vi "VT4001_Chamber Test.vi"(8 "error in":errorcluster, 10 "Target Temp(°C)":dbl=25.0, 11 "COM VISA Resource":refnum<visa-resource-name>="COM6") -> (0 "error out":errorcluster, 2 "OK":bool=TRUE)   [LabVIEW 2019]
doc: "Modbus Comm Tester\n\nThis VI demonstrates the usage of the Modbus Master API for both TCP and Serial connections.\nIt is also a useful tool for testing communication with your modbus device. You can test different\ncommunication parameters and coil/register address ranges without having to write any code.\n\nCopyright (c) 2016, Plasmionique Inc.\nAll rights reserved.\n\nLicense: BSD (2-Clause) - http://opensource.org/licenses/BSD-2-Clause"
uses:
  <vilib>/Plasmionique/MB Master/MB_Master_Serial/MB_Master_Serial.lvclass
  D:/National Instruments/LabVIEW 2019/vi.lib/Plasmionique/MB Master/MB_Master/MB_Master.lvclass
  <vilib>/Plasmionique/MB Master/MB Master.lvlib
panel:
  out "Numeric":i32
  out "Temp Read":u16
  # "Communication Settings"
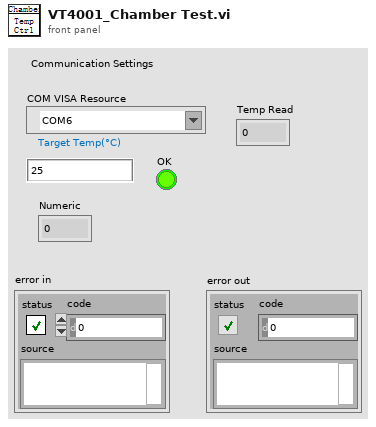
[diagram p1: front panel]
types:
  T1 = cluster{"baud rate (bps)":u32, "stop bits":u16, "parity":u16, "flow control":u16, "timeout":u32, "retries":i32}
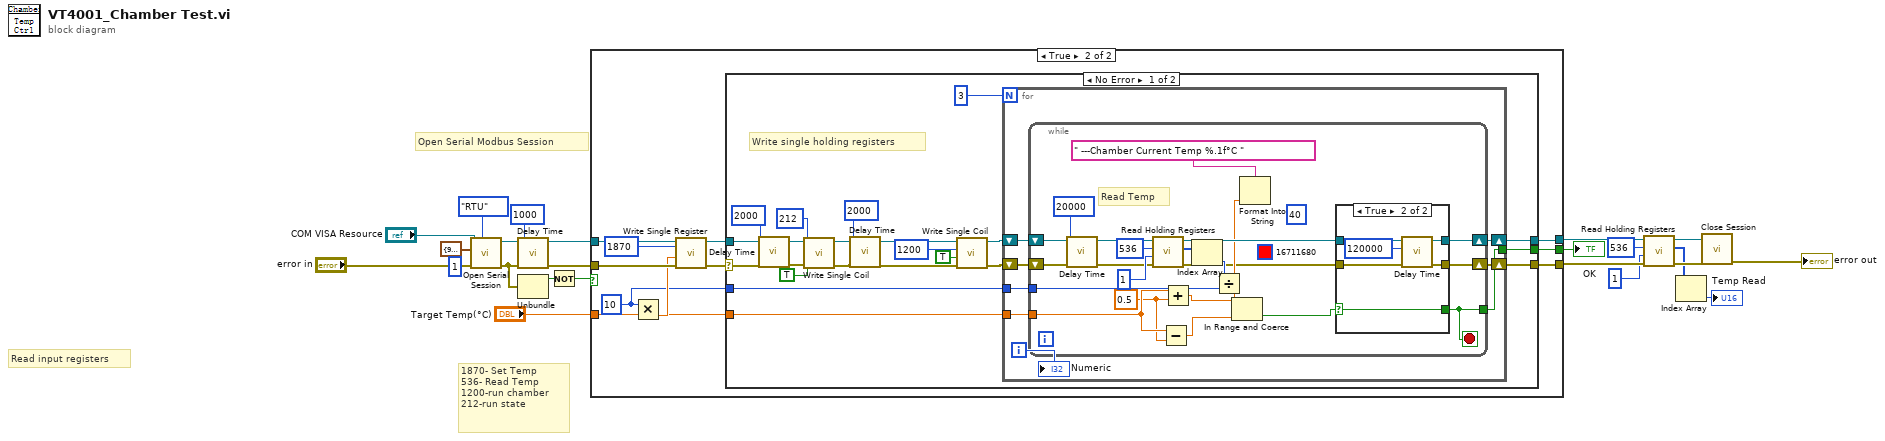
[diagram p0: block diagram]
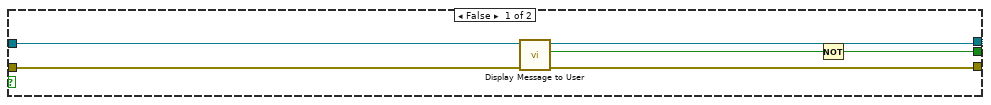
[diagram p2: hidden frame]
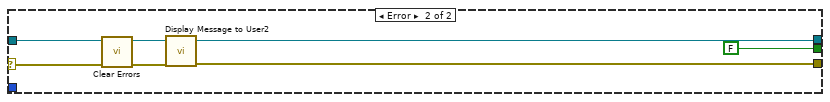
[diagram p4: hidden frame]
diagram:
  # "Open Serial Modbus Session"
  # "1870- Set Temp\n536- Read Temp\n1200-run chamber\n212-run state"
  # "Read input registers"
  n1 = call <vilib>:"Open Serial Session.vi"("Mode (RTU)"=enum16{"RTU", "ASCII"}."RTU", "Error in"="error in", "Slave ID"=u8 1, "Serial Config"=T1 {"baud rate (bps)"=9600, "stop bits"=10, "parity"=0, "flow control"=0, "timeout"=1000, "retries"=1}, "VISA Resource"="COM VISA Resource") -> ("Error out"=w19:errorcluster, "MB_Serial session"=w20:refnum<class "MB_Master_Serial.lvclass">)  [unwired: 5 in]
  n2 = call "Delay Time.vi"("Error In"=w19, "Delay Time (ms)"=u32 1000) -> ("Error Out"=w18:errorcluster)  [unwired: 9 in]
  n3 = Unbundle(w19) -> ("status"=w22:bool)  [unwired: 2 out]
  n4 = Not(x=w22) -> (.not. x?=w21:bool)
  n5 = case shown="True" w21 {
    tunnel: w20 -> [w23 w38]
    tunnel: w18 -> [w27 w37]
    tunnel: "Target Temp(°C)" -> [_ w29]
    tunnel: [w26 w36] -> w8
    tunnel: [w24 w35] -> w17
    tunnel: [w23 w34] -> w7
    frame False {
      n6 = call "Display Message to User"("error in (no error)"=w27) -> ("error out"=w26:errorcluster, "OK"=w25:bool)  [unwired: 9 in]
      n7 = Not(x=w25) -> (.not. x?=w24:bool)
    }
    frame True {
      w30 = u16 10 ("x")
      n8 = Multiply(x=w30, y=w29) -> (x*y=w31:dbl)
      n9 = call <vilib>:"Write Single Register.vi"("error in (no error)"=w37, "value"=w31, "address"=u16 1870, "MB session in"=w38) -> ("error out"=w28:errorcluster, "MB session out"=w32:refnum<class "MB_Master_Serial.lvclass">)  [unwired: 6 in]
      n10 = case shown="No Error" w28 {
        selector: w28 -> [w41 w96]
        tunnel: [w58 w98] -> w36
        tunnel: [w57 FALSE] -> w35
        tunnel: [w56 w100] -> w34
        tunnel: w32 -> [w46 w100]
        tunnel: w30 -> [w49 _]
        tunnel: w29 -> [w48 _]
        frame No Error {
          # "Write single holding registers"
          n11 = call "Delay Time.vi"("Error In"=w41, "Delay Time (ms)"=u32 2000) -> ("Error Out"=w45:errorcluster)  [unwired: 9 in]
          n12 = call <vilib>:"Write Single Coil.vi"("error in (no error)"=w45, "value"=TRUE, "address"=u16 212, "MB session in"=w46) -> ("error out"=w43:errorcluster, "MB session out"=w44:refnum<class "MB_Master_Serial.lvclass">)  [unwired: 6 in]
          n13 = call "Delay Time.vi"("Error In"=w43, "Delay Time (ms)"=u32 2000) -> ("Error Out"=w50:errorcluster)  [unwired: 9 in]
          n14 = call <vilib>:"Write Single Coil.vi"("error in (no error)"=w50, "value"=TRUE, "address"=u16 1200, "MB session in"=w44) -> ("error out"=w52:errorcluster, "MB session out"=w53:refnum<class "MB_Master_Serial.lvclass">)  [unwired: 6 in]
          n15 = for {
            N: 3 -> [_]
            tunnel: [w65] -> w57
            tunnel: w49 -> [w61]
            tunnel: w48 -> [w60]
            shift-right: [w64] -> w56
            shift-left: w53 -> [w63]
            shift-right: [w66] -> w58
            shift-left: w52 -> [w62]
            i -> [w59]
            n16 = while {
              tunnel: w60 -> [w77]
              tunnel: [w70] -> w65
              shift-right: [w86] -> w64
              shift-left: w63 -> [w84]
              shift-right: [w87] -> w66
              shift-left: w62 -> [w83]
              tunnel: w61 -> [w71]
              stop <- w70 stop-if-true
              (unwired) u32 40 ("Text.Font:Size")
              (unwired) u32 16711680 ("Color Box")
              w76 = 0.5
              # "Read Temp"
              n17 = call "Delay Time.vi"("Error In"=w83, "Delay Time (ms)"=u32 20000) -> ("Error Out"=w82:errorcluster)  [unwired: 9 in]
              n18 = call <vilib>:"Read Holding Registers.vi"("error in (no error)"=w82, "quantity"=u16 1, "starting address"=u16 536, "MB session in"=w84) -> ("error out"=w67:errorcluster, "Registers"=w81:u16[], "MB session out"=w79:refnum<class "MB_Master_Serial.lvclass">)  [unwired: 5 in]
              n19 = Subtract(x=w77, y=w76) -> (x-y=w73:dbl)
              n20 = Add(x=w77, y=w76) -> (x+y=w74:dbl)
              n21 = Index Array(array=w81) -> (element=w75:u16)  [unwired: 1 in]
              n22 = Divide(x=w75, y=w71) -> (x/y=w68:dbl)
              n23 = In Range and Coerce(upper limit=w74, x=w68, lower limit=w73) -> (In Range?=w72:bool)  [unwired: 1 out]
              n24 = Format Into String(format string=" ---Chamber Current Temp %.1f°C " ("string"), w68) -> ()  [unwired: 2 in, 2 out]
              n25 = case shown="True" w72 {
                selector: w72 -> [w90 w95]
                tunnel: [w90 w95] -> w70
                tunnel: w67 -> [w89 w94]
                tunnel: [w89 w93] -> w87
                tunnel: w79 -> [w88 w92]
                tunnel: [w88 w92] -> w86
                frame False {
                }
                frame True {
                  n26 = call "Delay Time.vi"("Error In"=w94, "Delay Time (ms)"=u32 120000) -> ("Error Out"=w93:errorcluster)  [unwired: 9 in]
                }
              }
            }
            "Numeric" <- w59
          }
        }
        frame Error {
          n27 = call <vilib>:"Clear Errors.vi"("error in (no error)"=w96) -> ("error out"=w97:errorcluster)  [unwired: 5 in, 1 out]
          n28 = call "Display Message to User2"("error in (no error)"=w97) -> ("error out"=w98:errorcluster)  [unwired: 9 in, 1 out]
        }
      }
    }
  }
  "OK" <- w17
  n29 = call <vilib>:"Read Holding Registers.vi"("error in (no error)"=w8, "quantity"=u16 1, "starting address"=u16 536, "MB session in"=w7) -> ("error out"=w5:errorcluster, "Registers"=w2:u16[], "MB session out"=w4:refnum<class "MB_Master_Serial.lvclass">)  [unwired: 5 in]
  n30 = Index Array(array=w2) -> (element=→"Temp Read":u16)  [unwired: 1 in]
  n31 = call-dynamic "Close Session.vi"("error in (no error)"=w5, "MB_Serial session"=w4) -> ("error out"=→"error out":errorcluster)  [unwired: 9 in]
